vi "SimulateIonImage.vi"(7 "Enum":T1(ring), 10 "height":i32=7, 11 "width":i32=15) -> (3 "Intensity Graph":i32[][](graph))   [LabVIEW 2019]
uses:
  <vilib>/gmath/statdist.llb/Normal PDF.vi
  <vilib>/gmath/NI_Gmath.lvlib
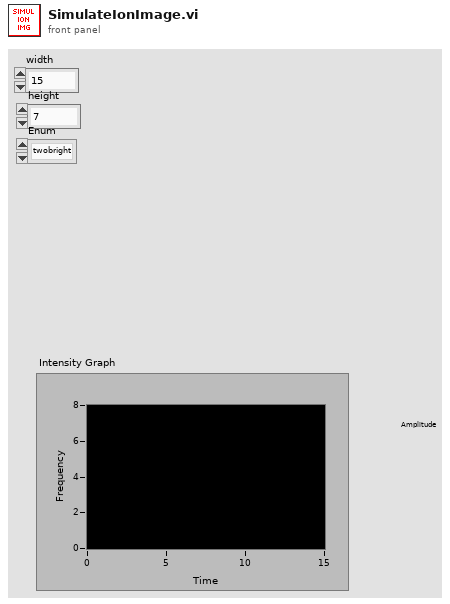
[diagram p1: front panel]
types:
  T1 = enum16{"twobright", "rightbright", "leftbright", "dark"}
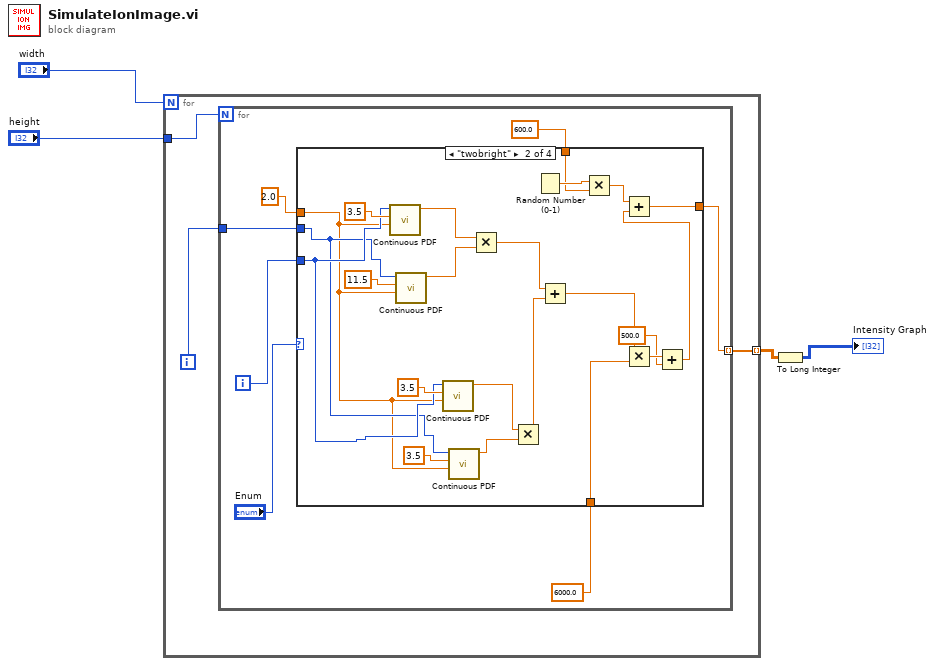
[diagram p0: block diagram]
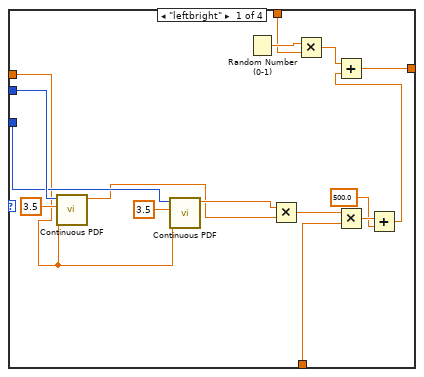
[diagram p2: hidden frame]
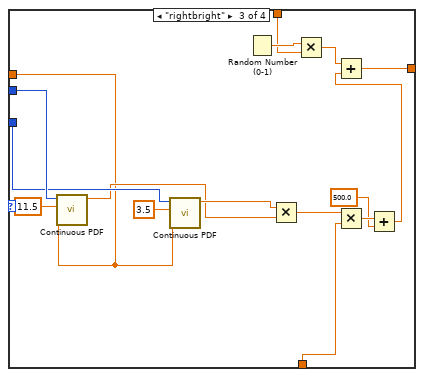
[diagram p3: hidden frame]
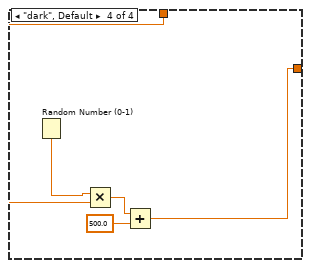
[diagram p4: hidden frame]
diagram:
  n1 = for {
    N: "width" -> [_]
    tunnel: [w6] -> w3 mode=indexing
    tunnel: "height" -> [w5]
    i -> [w7]
    n2 = for {
      N: w5 -> [_]
      tunnel: w7 -> [w14]
      tunnel: [w12] -> w6 mode=indexing
      i -> [w13]
      n3 = case shown="\"twobright\"" "Enum" {
        tunnel: w14 -> [w28 w39 w66 _]
        tunnel: w13 -> [w27 w40 w65 _]
        tunnel: [w18 w43 w56 w70] -> w12
        tunnel: 600.0 ("y") -> [w17 w33 w55 w69]
        tunnel: 6000.0 ("y") -> [w16 w32 w54 _]
        tunnel: 2.0 ("std") -> [w15 w31 w53 _]
        frame "leftbright" {
          n4 = call-poly <vilib>:"Continuous PDF.vi"("std"=w15, "mean"=3.5, "x"=w28) -> ("pdf(x)"=w25:dbl)  [unwired: 7 in, 1 out]
          n5 = call-poly <vilib>:"Continuous PDF.vi"("std"=w15, "mean"=3.5, "x"=w27) -> ("pdf(x)"=w26:dbl)  [unwired: 7 in, 1 out]
          n6 = Random Number (0-1)() -> (number: 0 to 1=w21:dbl)
          n7 = Multiply(x=w26, y=w25) -> (x*y=w24:dbl)
          n8 = Multiply(x=w21, y=w17) -> (x*y=w19:dbl)
          n9 = Multiply(x=w24, y=w16) -> (x*y=w23:dbl)
          n10 = Add(x=w23, y=500.0) -> (x+y=w20:dbl)
          n11 = Add(x=w19, y=w20) -> (x+y=w18:dbl)
        }
        frame "twobright" {
          n12 = call-poly <vilib>:"Continuous PDF.vi"("std"=w31, "mean"=3.5, "x"=w40) -> ("pdf(x)"=w50:dbl)  [unwired: 7 in, 1 out]
          n13 = call-poly <vilib>:"Continuous PDF.vi"("std"=w31, "mean"=11.5, "x"=w39) -> ("pdf(x)"=w49:dbl)  [unwired: 7 in, 1 out]
          n14 = call-poly <vilib>:"Continuous PDF.vi"("std"=w31, "mean"=3.5, "x"=w40) -> ("pdf(x)"=w37:dbl)  [unwired: 7 in, 1 out]
          n15 = call-poly <vilib>:"Continuous PDF.vi"("std"=w31, "mean"=3.5, "x"=w39) -> ("pdf(x)"=w38:dbl)  [unwired: 7 in, 1 out]
          n16 = Multiply(x=w50, y=w49) -> (x*y=w35:dbl)
          n17 = Multiply(x=w37, y=w38) -> (x*y=w36:dbl)
          n18 = Random Number (0-1)() -> (number: 0 to 1=w46:dbl)
          n19 = Add(x=w35, y=w36) -> (x+y=w34:dbl)
          n20 = Multiply(x=w46, y=w33) -> (x*y=w44:dbl)
          n21 = Multiply(x=w34, y=w32) -> (x*y=w48:dbl)
          n22 = Add(x=w48, y=500.0) -> (x+y=w45:dbl)
          n23 = Add(x=w44, y=w45) -> (x+y=w43:dbl)
        }
        frame "rightbright" {
          n24 = call-poly <vilib>:"Continuous PDF.vi"("std"=w53, "mean"=11.5, "x"=w66) -> ("pdf(x)"=w63:dbl)  [unwired: 7 in, 1 out]
          n25 = call-poly <vilib>:"Continuous PDF.vi"("std"=w53, "mean"=3.5, "x"=w65) -> ("pdf(x)"=w64:dbl)  [unwired: 7 in, 1 out]
          n26 = Random Number (0-1)() -> (number: 0 to 1=w59:dbl)
          n27 = Multiply(x=w64, y=w63) -> (x*y=w62:dbl)
          n28 = Multiply(x=w59, y=w55) -> (x*y=w57:dbl)
          n29 = Multiply(x=w62, y=w54) -> (x*y=w61:dbl)
          n30 = Add(x=w61, y=500.0) -> (x+y=w58:dbl)
          n31 = Add(x=w57, y=w58) -> (x+y=w56:dbl)
        }
        frame "dark", Default {
          n32 = Random Number (0-1)() -> (number: 0 to 1=w73:dbl)
          n33 = Multiply(x=w73, y=w69) -> (x*y=w72:dbl)
          n34 = Add(x=w72, y=500.0) -> (x+y=w70:dbl)
        }
      }
    }
  }
  n35 = To Long Integer(number=w3) -> (32bit integer=→"Intensity Graph":i32[][])
